vi "Build Variability Plot from Reference.vi"(4 "Group Cols":i32[](array[numeric])=[2], 6 "Y-axis Col":i32=20, 8 "Size of Legend (%)":dbl=0.2, 9 "Column Header Strings":string[](array[string])=["Unique_ID", "Wafer_Name", "Split", "Cell", "Sample_Type", "Experiment", "Active_Area_(cm2)", "Num_of_cell_tests", "Date-Time", "User_Name", "Irradiance_(W/cm2)", "Temperature(C)", "Sweep_Type", "Bulb_Power", "Bulb_Flux(uA)", "Last_Calibrated_Date-Time", "Last_Bulb_Replacement_Date-Time", "Comments", "Unique_ID", "Eff", "Voc_(V)", "Jsc_(A/cm2)", "Fill_Factor", "Roc_(ohm*cm2)", "Rsc_(ohm*cm2)", "Pmax_(W/cm2)", "Vmp_(V)", "Jmp_(A/cm2)", "Model R2", "Dark_Turn-on_V", "Ideality_Factor", "J0_(A/cm2)", "J0_Diffusion_(A/cm2)", "J0_GR_(A/cm2)", "Rsh_(Ohm*cm2)", "Rs_(Ohm*cm2)", "CE_(%)"], 10 "Input Table":string[][](array[string])=[["ID03172011132910", "D11014", "B5", "1", "Crystal CdTe", "CZT EXP009", "0.0143", "2", "3/17/2011 1:29:10 PM", "dtester", "0.1", "25", "Custom - Uses option tab setting", "1155", "161.6", "3/17/2011 1:24:56 PM", "5/25/2010 1:00:00 PM", "", "ID03172011132910", "0.000018331135", "0.329199646", "-0.000019162902", "0.290582012", "12248.694", "23122.247", "0.000001833114", "0.179016841", "0.000010239894", "0", "0.992889686", "8.68126209E-46", "4.422637E-12", "4451299", "-131.960127", "61928.868", "", "", "", "", ""], ["ID03172011133056", "D11014", "B5", "2", "Crystal CdTe", "CZT EXP009", "0.0143", "1", "3/17/2011 1:30:56 PM", "dtester", "0.1", "25", "Custom - Uses option tab setting", "1155", "161.6", "3/17/2011 1:24:56 PM", "5/25/2010 1:00:00 PM", "", "ID03172011133056", "0.000019774033", "0.343694416", "-0.000019403825", "0.29650732", "11605.468", "24816.221", "0.000001977403", "0.188833978", "0.00001047165", "3222.311", "0.992305147", "4.10762544E-46", "4.64417E-12", "5095988", "-116.319344", "80376.492", "", "", "", "", ""], ["ID03172011134450", "D11016", "E4", "1", "Crystal CdTe", "CZT EXP009", "0.0143", "2", "3/17/2011 1:44:50 PM", "dtester", "0.1", "25", "Custom - Uses option tab setting", "0", "161.6", "3/17/2011 1:24:56 PM", "5/25/2010 1:00:00 PM", "", "ID03172011134450", "0", "0.066337846", "-0.000001549743", "0", "24000.955", "355279.503", "0", "0", "0", "0", "0.932694566", "4.712838E-48", "1.521848E-12", "100000000000000", "-1301.062", "361382.131", "", "", "", "", ""], ["ID03172011134552", "D11016", "E4", "2", "Crystal CdTe", "CZT EXP009", "0.0143", "1", "3/17/2011 1:45:52 PM", "dtester", "0.1", "25", "Custom - Uses option tab setting", "0", "161.6", "3/17/2011 1:24:56 PM", "5/25/2010 1:00:00 PM", "", "ID03172011134552", "0.000001609791", "0.18902661", "-0.000004209879", "0.202291173", "55653.293", "29563.168", "0.0000001609791", "0.093729707", "0.000001717482", "0", "0.836775618", "3.606545E-48", "0.000000003769194", "100000000000000", "-504.246188", "546040.796", "", "", "", "", ""], ["ID03172011134725", "D11017", "A3", "1", "Crystal CdTe", "CZT EXP009", "0.0143", "1", "3/17/2011 1:47:25 PM", "dtester", "0.1", "25", "Custom - Uses option tab setting", "0", "161.6", "3/17/2011 1:24:56 PM", "5/25/2010 1:00:00 PM", "", "ID03172011134725", "0.000007862703", "0.300634425", "-0.000009351238", "0.279681693", "25122.784", "37448.672", "0.00000078627026", "0.161786792", "0.000004859916", "0", "0.998501747", "1.881718E-48", "3.03841765E-10", "7111744", "-173.547592", "554111.9", "", "", "", "", ""], ["ID03172011134847", "D11017", "A3", "3", "Crystal CdTe", "CZT EXP009", "0.0143", "1", "3/17/2011 1:48:47 PM", "dtester", "0.1", "25", "Custom - Uses option tab setting", "0", "161.6", "3/17/2011 1:24:56 PM", "5/25/2010 1:00:00 PM", "", "ID03172011134847", "0.000007726846", "0.299639907", "-0.000009106517", "0.283171979", "25227.847", "39025.402", "0.000000772684597", "0.161170617", "0.000004794203", "29301660", "0.996689983", "9.30590943E-49", "8.7875222E-11", "7981629", "-169.139745", "676093.501", "", "", "", "", ""], ["ID03172011135004", "D11016", "E2", "1", "Crystal CdTe", "CZT EXP009", "0.0143", "1", "3/17/2011 1:50:04 PM", "dtester", "0.1", "25", "Custom - Uses option tab setting", "0", "161.6", "3/17/2011 1:24:56 PM", "5/25/2010 1:00:00 PM", "", "ID03172011135004", "0.000008887575", "0.314422094", "-0.000011008741", "0.256763078", "24162.056", "38566.512", "0.000000888757533", "0.135568669", "0.000006555774", "372634.151", "0.99877204", "2.5938593E-47", "1.00830354E-10", "6315776", "-188.727106", "224030.183", "", "", "", "", ""], ["ID03172011135102", "D11016", "E2", "2", "Crystal CdTe", "CZT EXP009", "0.0143", "1", "3/17/2011 1:51:02 PM", "dtester", "0.1", "25", "Custom - Uses option tab setting", "0", "161.6", "3/17/2011 1:24:56 PM", "5/25/2010 1:00:00 PM", "", "ID03172011135102", "0.000008220737", "0.299774635", "-0.000008826217", "0.310700021", "23973.842", "26397.011", "0.000000822073702", "0.180441307", "0.000004555906", "0", "0.998383932", "2.0025352E-47", "1.04854738E-10", "6274781", "-214.846448", "244423.023", "", "", "", "", ""], ["ID03172011135230", "D11017", "C1", "1", "Crystal CdTe", "CZT EXP009", "0.0143", "1", "3/17/2011 1:52:30 PM", "dtester", "0.1", "25", "Custom - Uses option tab setting", "0", "161.6", "3/17/2011 1:24:56 PM", "5/25/2010 1:00:00 PM", "", "ID03172011135230", "0.000009002015", "0.322095736", "-0.000010017559", "0.278992685", "25552.404", "38853.628", "0.000000900201474", "0.172166433", "0.00000522867", "16809035", "0.998577656", "5.83859492E-49", "3.0578151E-10", "7303523", "-156.257879", "798891.399", "", "", "", "", ""], ["ID03172011135446", "D11014", "A2", "1", "Crystal CdTe", "CZT EXP009", "0.0143", "1", "3/17/2011 1:54:46 PM", "dtester", "0.1", "25", "Custom - Uses option tab setting", "0", "161.6", "3/17/2011 1:24:56 PM", "5/25/2010 1:00:00 PM", "retry", "ID03172011135446", "0.000008121558", "0.318938896", "-0.000008607329", "0.295844468", "25228.235", "29753.235", "0.000000812155756", "0.158334247", "0.000005129375", "0", "0.996400609", "2.016331E-48", "3.99575382E-10", "9290112", "-74.919625", "546763.331", "", "", "", "", ""], ["ID03172011135542", "D11014", "A2", "2", "Crystal CdTe", "CZT EXP009", "0.0143", "1", "3/17/2011 1:55:42 PM", "dtester", "0.1", "25", "Custom - Uses option tab setting", "0", "162", "3/17/2011 1:24:56 PM", "5/25/2010 1:00:00 PM", "retry", "ID03172011135542", "0.000010769773", "0.316532242", "-0.000010678727", "0.31861711", "18332.836", "32777.717", "0.000001076977", "0.185023821", "0.000005820749", "0", "0.994541054", "3.879299E-48", "9.0565763E-11", "8933675", "-113.837654", "437235.26", "", "", "", "", ""], ["ID03172011135702", "D11016", "C3", "1", "Crystal CdTe", "CZT EXP009", "0.0143", "1", "3/17/2011 1:57:02 PM", "dtester", "0.1", "25", "Custom - Uses option tab setting", "0", "161.6", "3/17/2011 1:24:56 PM", "5/25/2010 1:00:00 PM", "retry", "ID03172011135702", "0.000005099675", "0.235096132", "-0.000007926189", "0.27367339", "25734.358", "34044.701", "0.000000509967465", "0.123146343", "0.00000414115", "4091317000", "0.989780648", "6.5732986E-50", "0.00000012792339", "6862941", "-258.957329", "1691082", "", "", "", "", ""], ["ID03172011135800", "D11016", "C3", "2", "Crystal CdTe", "CZT EXP009", "0.0143", "1", "3/17/2011 1:58:00 PM", "dtester", "0.1", "25", "Custom - Uses option tab setting", "0", "161.6", "3/17/2011 1:24:56 PM", "5/25/2010 1:00:00 PM", "retry", "ID03172011135800", "0.000006572242", "0.277556032", "-0.00000897193", "0.263922873", "36049.094", "36545.224", "0.000000657224249", "0.14400509", "0.000004563896", "4327975000000", "0.969663856", "1.11030837E-52", "3.012567E-14", "205688100", "-168.692902", "9146911", "", "", "", "", ""]], 11 "Variability Plot Reference":refnum<vi>) -> ()   [LabVIEW 2010]
uses:
  <vilib>/Analysis/NI_AALBase.lvlib
panel:
  out "appended array":cluster{dbl[], dbl[]}[](array[cluster])
  out "subarray":dbl[](array[numeric])
  out "Bottom":dbl=0.010866531999999998
  out "Array":cluster{"String":string, dbl, dbl}[](array[cluster])=[{"String"="A2", 1.0, 0.038602189}, {"String"="A3", 2.0, 0.038602189}, {"String"="B5", 3.0, 0.038602189}, {"String"="C1", 4.0, 0.038602189}, {"String"="C3", 5.0, 0.038602189}, {"String"="E2", 6.0, 0.038602189}, {"String"="E4", 7.0, 0.038602189}]
  out "List of Categories":string[][](array[string])=[["A2"], ["A3"], ["B5"], ["C1"], ["C3"], ["E2"], ["E4"]]
  out "Parameter Analysis Graph":cluster{"Voltage":dbl[], dbl[]}[](graph)=[{"Voltage"=[3.0, 3.0, 7.0, 7.0, 2.0, 2.0, 6.0, 6.0, 4.0, 1.0, 1.0, 5.0, 5.0], [0.329199646, 0.343694416, 0.066337846, 0.18902661, 0.300634425, 0.299639907, 0.314422094, 0.299774635, 0.322095736, 0.318938896, 0.316532242, 0.235096132, 0.277556032]}, {"Voltage"=[1.0, 2.0, 3.0, 4.0, 5.0, 6.0, 7.0], [0.317735569, 0.30013716599999996, 0.336447031, 0.322095736, 0.256326082, 0.3070983645, 0.127682228]}, {"Voltage"=[0.0, 8.0, 8.0, 0.0], [0.010866531999999998, 0.010866531999999998, 0.066337846, 0.066337846]}, {"Voltage"=[0.5, 0.5], [0.066337846, inf]}]
  # "Most General"
  # "Most Specific"
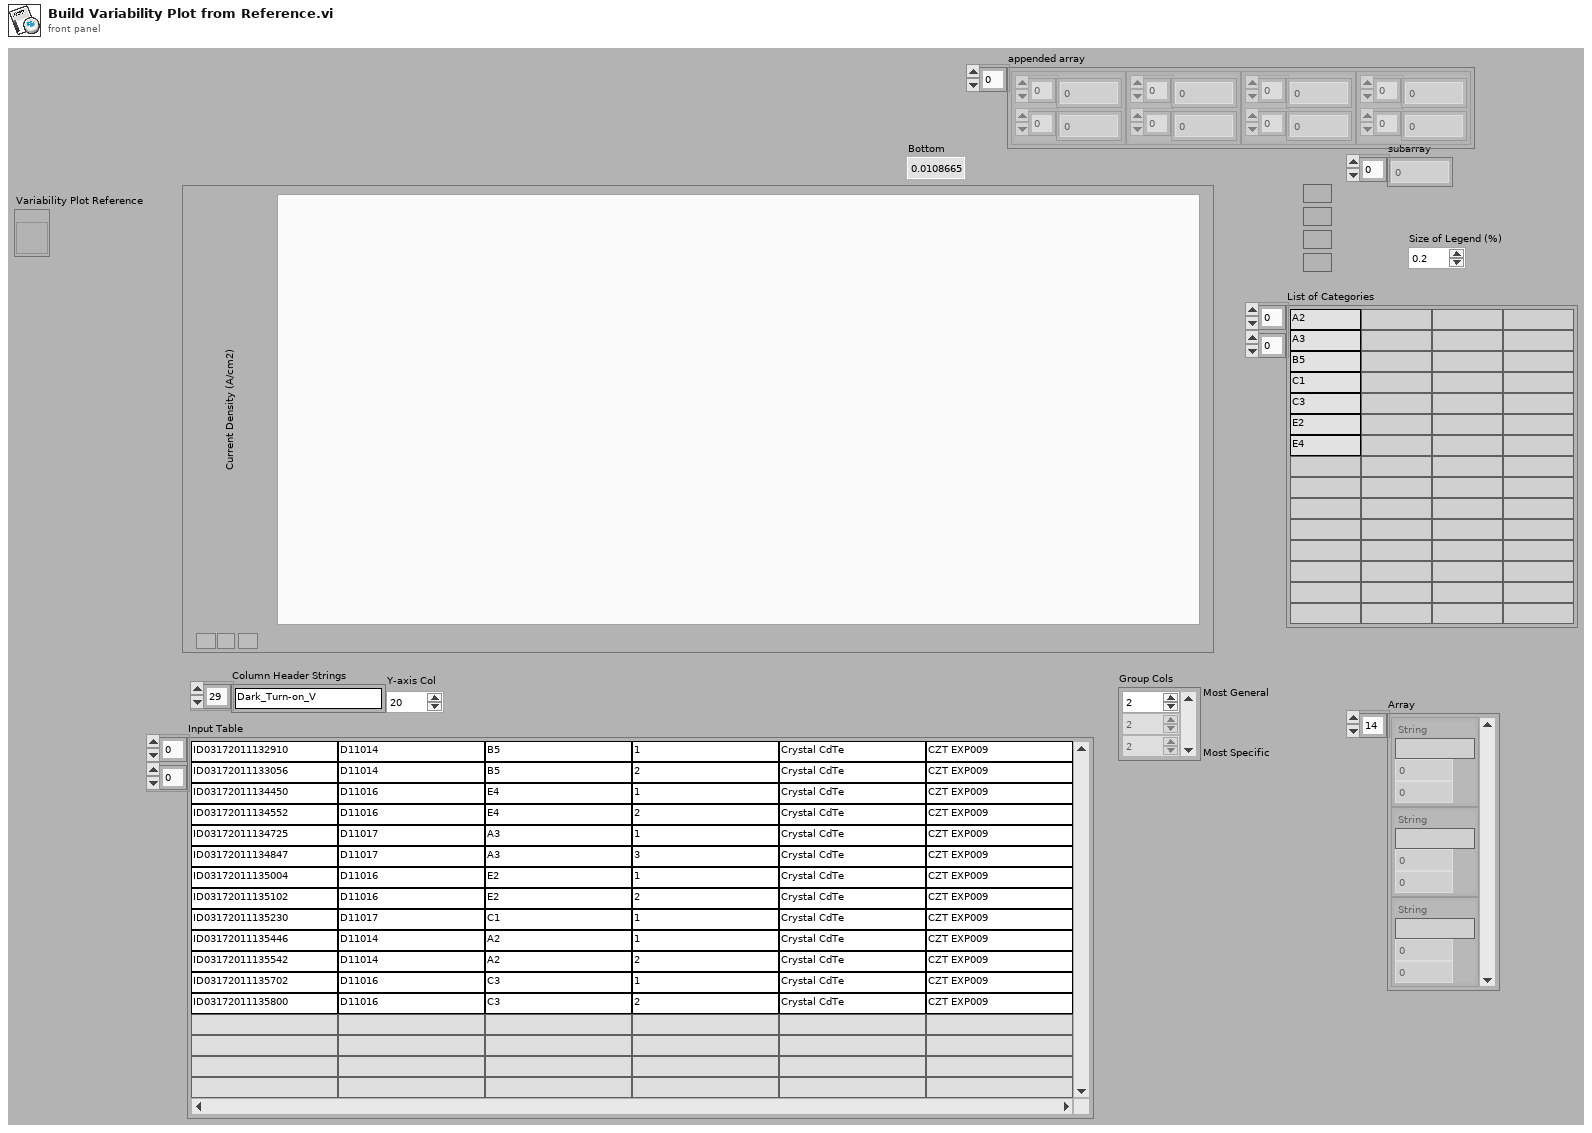
[diagram p1: front panel]
types:
  T1 = cluster{"Name":string, "Color":u32, "Style":u8, "Point Style":u8, "Name Visible":bool, "Allow Drag":bool, "Annotation Mode":u32, "Plot":i32, "Index":i32, "Position":cluster{"X":dbl, "Y":dbl}, "X Scale":u32, "Y Scale":u32, "Show Arrow":bool, "Lock Name":bool, "Plot Area":i32, "Label Offset":cluster{"X":dbl, "Y":dbl}}
  T2 = cluster{"Name":string, "Color":u32, "Style":u8, "Point Style":u8, "Name Visible":bool, "Allow Drag":bool, "Annotation Mode":u32, "Plot":i32, "Index":i32, "Position":cluster{"X":dbl, "Y":dbl}, "X Scale":u32, "Y Scale":u32, "Show Arrow":bool, "Lock Name":bool, "Plot Area":i32, "Label Offset":cluster{"X":dbl, "Y":dbl}}[]
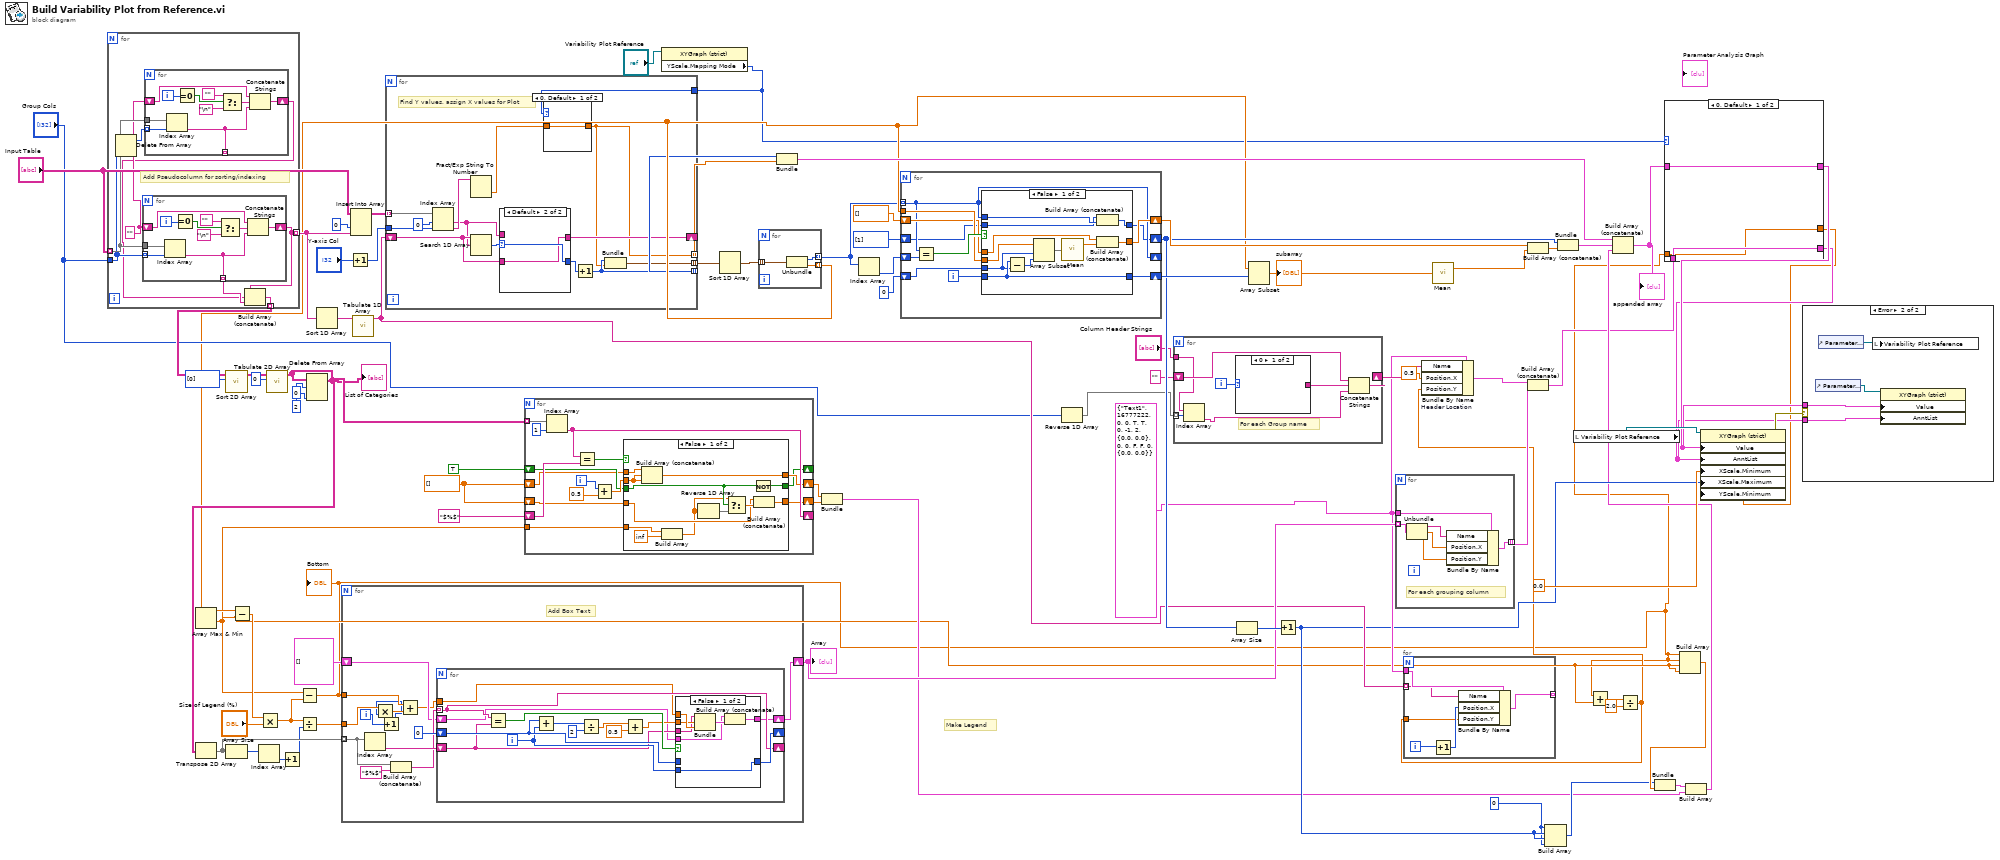
[diagram p0: block diagram]
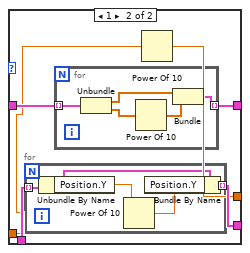
[diagram p2: hidden frame]
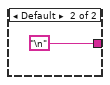
[diagram p6: hidden frame]
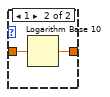
[diagram p8: hidden frame]
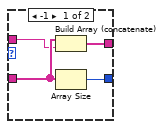
[diagram p9: hidden frame]
diagram:
  w27 = 0
  w46 = dbl[] []
  w29 = T1 {"Name"="Text1", "Color"=16777222, "Style"=0, "Point Style"=0, "Name Visible"=TRUE, "Allow Drag"=TRUE, "Annotation Mode"=0, "Plot"=-1, "Index"=2, "Position"={"X"=0.0, "Y"=0.0}, "X Scale"=0, "Y Scale"=0, "Show Arrow"=FALSE, "Lock Name"=FALSE, "Plot Area"=0, "Label Offset"={"X"=0.0, "Y"=0.0}} ("element")
  # "Make Legend"
  n1 = for {
    tunnel: "Input Table" -> [w87] mode=indexing
    tunnel: "Group Cols" -> [w85]
    tunnel: [w90] -> w64 mode=indexing
    tunnel: [w88] -> w52 mode=indexing
    w86 = ""
    # "Add Pseudocolumn for sorting/indexing"
    n2 = Delete From Array(array=w85) -> (array with subset deleted=w84:i32[])  [unwired: 2 in, 1 out]
    n3 = for {
      tunnel: w85 -> [w109] mode=indexing
      tunnel: w87 -> [w110]
      shift-right: [w108] -> w90
      shift-left: w86 -> [w107]
      tunnel: [w101] -> w89 mode=indexing
      i -> [w105]
      n4 = Index Array(array=w110, index=w109) -> (element=w101:string)
      n5 = Equal To 0?(x=w105) -> (x = 0?=w106:bool)
      n6 = Select(t="", s=w106, f="\n") -> (s? t:f=w102:string)
      n7 = Concatenate Strings(w107, w102, w101) -> (w108:string)
    }
    n8 = for {
      tunnel: w84 -> [w99] mode=indexing
      tunnel: w87 -> [w100]
      shift-right: [w98] -> w83
      shift-left: w86 -> [w97]
      tunnel: [w91] -> _ mode=indexing
      i -> [w95]
      n9 = Index Array(array=w100, index=w99) -> (element=w91:string)
      n10 = Equal To 0?(x=w95) -> (x = 0?=w96:bool)
      n11 = Select(t="", s=w96, f="\n") -> (s? t:f=w92:string)
      n12 = Concatenate Strings(w97, w92, w91) -> (w98:string)
    }
    n13 = Build Array (concatenate)(w90, w83, w89) -> (w88:string[])
  }
  n14 = call "Sort 2D Array.vi"("Sort by Cols"=i32[] [0], "Input Array"=w52) -> ("Output Array"=w55:string[][])  [unwired: 9 in]
  n15 = call "Tabulate 2D Array.vi"("Tabulation Column"=0, "Input Array"=w55) -> ("Tabulation"=w42:string[][])  [unwired: 9 in]
  n16 = Delete From Array(array=w42, length=2, index (col)=0 ("index (row)")) -> (array with subset deleted=w41:string[][])  [unwired: 1 in, 1 out]
  "List of Categories" <- w41
  n17 = Transpose 2D Array(2D array=w41) -> (transposed array=w34:string[][])
  n18 = Array Size(array=w34) -> (size(s)=w33:i32[])
  n19 = Index Array(array=w33) -> (element=w20:i32)  [unwired: 1 in]
  n20 = Increment(x=w20) -> (x+1=w19:i32)
  n21 = Sort 1D Array(array=w64) -> (sorted array=w67:string[])
  n22 = Increment(x="Y-axis Col") -> (x+1=w63:i32)
  n23 = Insert Into Array(array="Input Table", index (col)=0 ("disabled index (col)"), new element=w64) -> (w57:string[][])  [unwired: 1 in]
  n24 = call "Tabulate 1D Array.vi"("1D Array"=w67) -> ("Tabulated Array"=w39:string[])  [unwired: 10 in]
  n25 = property class="XYGraph (strict)"(reference="Variability Plot Reference") -> ("YScale.Mapping Mode"=w1:u8)  [unwired: 1 in, 2 out]
  n26 = for {
    tunnel: w57 -> [w119] mode=indexing
    shift-right: [w123] -> _
    shift-left: w39 -> [w122]
    tunnel: [w111] -> w2 mode=indexing
    tunnel: [w120] -> w66 mode=indexing
    tunnel: w63 -> [w118]
    tunnel: [w116] -> w3 mode=indexing
    tunnel: w1 -> [w113]
    # "Find Y values, assign X values for Plot"
    n27 = Index Array(array=w119, index #1=0 ("index"), index #2=w118) -> (element #1=w115:string, element #2=w117:string)
    n28 = Fract/Exp String To Number(string=w117) -> (number=w112:dbl)  [unwired: 3 in, 1 out]
    n29 = Search 1D Array(1D array=w122, element=w115) -> (index of element=w124:i32)  [unwired: 1 in]
    n30 = case shown="Default" w124 {
      selector: w124 -> [_ w133]
      tunnel: w115 -> [w128 _]
      tunnel: [w131 w132] -> w123
      tunnel: w122 -> [w129 w132]
      tunnel: [w130 w133] -> w121
      frame -1 {
        n31 = Build Array (concatenate)(w129, w128) -> (w131:string[])
        n32 = Array Size(array=w129) -> (size(s)=w130:i32)
      }
      frame Default {
      }
    }
    n33 = case shown="0, Default" w113 {
      tunnel: w112 -> [w125 w127]
      tunnel: [w125 w126] -> w111
      frame 0, Default {
      }
      frame 1 {
        n34 = Logarithm Base 10(1:w127) -> (0:w126:dbl)
      }
    }
    n35 = Increment(x=w121) -> (x+1=w116:i32)
    n36 = Bundle(w116, w111) -> (w120:cluster{i32, dbl})  [unwired: 1 in]
  }
  n37 = Sort 1D Array(array=w66) -> (sorted array=w59:cluster{i32, dbl}[])
  n38 = for {
    tunnel: w59 -> [w136] mode=indexing
    tunnel: [w135] -> w4 mode=indexing
    tunnel: [w134] -> w10 mode=indexing
    n39 = Unbundle(w136) -> (w135:i32, w134:dbl)
  }
  n40 = Array Max & Min(array=w10) -> (max value=w30:dbl, min value=w16:dbl)  [unwired: 2 out]
  n41 = Subtract(x=w30, y=w16) -> (x-y=w26:dbl)
  n42 = Multiply(x=w26, y="Size of Legend (%)") -> (x*y=w35:dbl)
  n43 = Subtract(x=w16, y=w35) -> (x-y=w7:dbl)
  "Bottom" <- w7
  n44 = Divide(x=w35, y=w19) -> (x/y=w32:dbl)
  n45 = for {
    tunnel: w34 -> [w147] mode=indexing
    shift-right: [w144] -> w40
    shift-left: cluster{"String":string, dbl, dbl}[] [] -> [w143]
    tunnel: w7 -> [w140]
    tunnel: w32 -> [w139]
    i -> [w138]
    # "Add Box Text"
    n46 = Index Array(array=w147) -> (element=w149:string)  [unwired: 1 in]
    n47 = Increment(x=w138) -> (x+1=w137:i32)
    n48 = Multiply(x=w139, y=w137) -> (x*y=w142:dbl)
    n49 = Build Array (concatenate)(w147, "$%$" ("String")) -> (w145:string[])
    n50 = Add(x=w140, y=w142) -> (x+y=w141:dbl)
    n51 = for {
      tunnel: w145 -> [w155] mode=indexing
      shift-right: [w155] -> _
      shift-left: w149 -> [w153]
      shift-right: [w162] -> _
      shift-left: 0 -> [w158]
      shift-right: [w151] -> w144
      shift-left: w143 -> [w150]
      tunnel: w141 -> [w152]
      i -> [w157]
      n52 = Equal?(x=w155, y=w153) -> (x = y?=w163:bool)
      n53 = Add(x=w158, y=w157) -> (x+y=w156:i32)
      n54 = Divide(x=w156, y=2) -> (x/y=w160:dbl)
      n55 = Add(x=w160, y=0.5) -> (x+y=w154:dbl)
      n56 = case shown="False" w163 {
        tunnel: w157 -> [w170 _]
        tunnel: [w170 w172] -> w162
        tunnel: w158 -> [_ w172]
        tunnel: w154 -> [w168 _]
        tunnel: w152 -> [w169 _]
        tunnel: w153 -> [w167 _]
        tunnel: [w165 w171] -> w151
        tunnel: w150 -> [w164 w171]
        frame False {
          n57 = Bundle("String"=w167, w168, w169) -> (w166:cluster{"String":string, dbl, dbl})  [unwired: 1 in]
          n58 = Build Array (concatenate)(w164, w166) -> (w165:cluster{"String":string, dbl, dbl}[])
        }
        frame True {
        }
      }
    }
  }
  "Array" <- w40
  n59 = for {
    tunnel: w42 -> [w187] mode=indexing
    shift-right: [w186] -> _
    shift-left: "$%$" ("String") -> [w185]
    shift-right: [w179] -> w45
    shift-left: w46 -> [w178]
    shift-right: [w177] -> _
    shift-left: TRUE -> [w180]
    shift-right: [w176] -> w44
    shift-left: w46 -> [w175]
    tunnel: w16 -> [w173]
    i -> [w183]
    n60 = Index Array(array=w187, index=1) -> (element=w186:string)
    n61 = Equal?(x=w186, y=w185) -> (x = y?=w184:bool)
    n62 = Add(x=w183, y=0.5) -> (x+y=w181:dbl)
    n63 = case shown="False" w184 {
      tunnel: w181 -> [w199 _]
      tunnel: w180 -> [w195 w202]
      tunnel: [w197 w200] -> w179
      tunnel: w178 -> [w196 w200]
      tunnel: [w194 w202] -> w177
      tunnel: [w192 w201] -> w176
      tunnel: w175 -> [w191 w201]
      tunnel: w173 -> [w189 _]
      frame False {
        n64 = Build Array (concatenate)(w196, w199, w199) -> (w197:dbl[])
        n65 = Build Array(w189, inf) -> (w188:dbl[])
        n66 = Reverse 1D Array(array=w188) -> (reversed array=w198:dbl[])
        n67 = Select(t=w188, s=w195, f=w198) -> (s? t:f=w193:dbl[])
        n68 = Not(x=w195) -> (.not. x?=w194:bool)
        n69 = Build Array (concatenate)(w191, w193) -> (w192:dbl[])
      }
      frame True {
      }
    }
  }
  n70 = Bundle(w3, w2) -> (w78:cluster{i32[], dbl[]})  [unwired: 1 in]
  n71 = Bundle(w45, w44) -> (w22:cluster{dbl[], dbl[]})  [unwired: 1 in]
  n72 = Index Array(array=w4) -> (element=w82:i32)  [unwired: 1 in]
  n73 = for {
    tunnel: w4 -> [w205] mode=indexing
    tunnel: w10 -> [w208]
    shift-right: [w205] -> _
    shift-left: w82 -> [w213]
    shift-right: [w210] -> w76
    shift-left: 0 -> [w209]
    shift-right: [w207] -> w74
    shift-left: dbl[] [] -> [w206]
    shift-right: [w204] -> w62
    shift-left: i32[] [1] -> [w203]
    i -> [w211]
    n74 = Equal?(x=w205, y=w213) -> (x = y?=w212:bool)
    n75 = case shown="False" w212 {
      tunnel: w211 -> [w223 _]
      tunnel: [w223 w227] -> w210
      tunnel: w209 -> [w222 w227]
      tunnel: w208 -> [w224 _]
      tunnel: [w220 w226] -> w207
      tunnel: w206 -> [w219 w226]
      tunnel: w205 -> [w218 _]
      tunnel: [w217 w225] -> w204
      tunnel: w203 -> [w216 w225]
      frame False {
        n76 = Subtract(x=w223, y=w222) -> (x-y=w221:i32)
        n77 = Array Subset(array=w224, index=w222, length=w221) -> (w215:dbl[])
        n78 = call <vilib>:"Mean.vi"("X"=w215) -> ("mean"=w214:dbl)  [unwired: 1 out]
        n79 = Build Array (concatenate)(w216, w218) -> (w217:i32[])
        n80 = Build Array (concatenate)(w219, w214) -> (w220:dbl[])
      }
      frame True {
      }
    }
  }
  n81 = Reverse 1D Array(array="Group Cols") -> (reversed array=w49:i32[])
  n82 = for {
    shift-right: [w233] -> w72
    shift-left: "" -> [w232]
    tunnel: "Column Header Strings" -> [w230]
    tunnel: w49 -> [w229] mode=indexing
    i -> [w231]
    # "For each Group name"
    n83 = Index Array(array=w230, index=w229) -> (element=w228:string)
    n84 = case shown="0" w231 {
      tunnel: [_ "\n"] -> w234
      frame 0 {
      }
      frame Default {
      }
    }
    n85 = Concatenate Strings(w232, w234, w228) -> (w233:string)
  }
  n86 = Array Size(array=w62) -> (size(s)=w68:i32)
  n87 = Array Subset(array=w10, index=w76) -> (w75:dbl[])  [unwired: 1 in]
  "subarray" <- w75
  n88 = Increment(x=w68) -> (x+1=w28:i32)
  n89 = for {
    tunnel: w29 -> [w241]
    tunnel: [w240] -> w69 mode=indexing
    tunnel: w40 -> [w239] mode=indexing
    # "For each grouping column"
    n90 = Unbundle(w239) -> ("String"=w238:string, w237:dbl, w236:dbl)
    n91 = Bundle By Name(cluster=w241, "Name"=w238, "Position.X"=w237, "Position.Y"=w236) -> (w240:T1)
  }
  n92 = call <vilib>:"Mean.vi"("X"=w75) -> ("mean"=w5:dbl)  [unwired: 1 out]
  n93 = Build Array (concatenate)(w74, w5) -> (w73:dbl[])
  n94 = Build Array(w27, w28, w28, w27) -> (w24:i32[])
  n95 = Bundle(w62, w73) -> (w79:cluster{i32[], dbl[]})  [unwired: 1 in]
  n96 = local read "Variability Plot Reference"() -> (w13:refnum<vi>)
  n97 = Add(x=w7, y=w16) -> (x+y=w18:dbl)
  n98 = Divide(x=w18, y=2.0) -> (x/y=w15:dbl)
  n99 = for {
    tunnel: w39 -> [w246] mode=indexing
    tunnel: w29 -> [w247]
    tunnel: [w243] -> _ mode=indexing
    tunnel: w15 -> [w242]
    i -> [w245]
    n100 = Increment(x=w245) -> (x+1=w244:i32)
    n101 = Bundle By Name(cluster=w247, "Name"=w246, "Position.X"=w244, "Position.Y"=w242) -> (w243:T1)
  }
  n102 = Bundle By Name "Header Location"(cluster=w29, "Name"=w72, "Position.X"=0.5, "Position.Y"=w15) -> (w70:T1)
  n103 = Build Array (concatenate)(w70, w69) -> (w9:T2)
  n104 = Build Array(w7, w7, w16, w16) -> (w25:dbl[])
  n105 = Bundle(w24, w25) -> (w23:cluster{i32[], dbl[]})  [unwired: 1 in]
  n106 = Build Array(w23, w22) -> (w21:cluster{dbl[], dbl[]}[])
  n107 = Build Array (concatenate)(w78, w79, w21) -> (w12:cluster{dbl[], dbl[]}[])
  "appended array" <- w12
  n108 = case shown="0, Default" w1 {
    tunnel: w12 -> [w250 w256]
    tunnel: [w250 w255] -> w11
    tunnel: w9 -> [w249 w254]
    tunnel: [w249 w253] -> w8
    tunnel: w7 -> [w248 w252]
    tunnel: [w248 w251] -> w6
    frame 0, Default {
    }
    frame 1 {
      n109 = for {
        tunnel: w254 -> [w260] mode=indexing
        tunnel: [w259] -> w253 mode=indexing
        n110 = Unbundle By Name(w260) -> ("Position.Y"=w258:dbl)
        n111 = Power Of 10(x=w258) -> (10^x=w257:dbl)
        n112 = Bundle By Name(cluster=w260, "Position.Y"=w257) -> (w259:T1)
      }
      n113 = for {
        tunnel: w256 -> [w265] mode=indexing
        tunnel: [w261] -> w255 mode=indexing
        n114 = Unbundle(w265) -> (w263:dbl[], w264:dbl[])
        n115 = Power Of 10(x=w264) -> (10^x=w262:dbl[])
        n116 = Bundle(w263, w262) -> (w261:cluster{dbl[], dbl[]})  [unwired: 1 in]
      }
      n117 = Power Of 10(x=w252) -> (10^x=w251:dbl)
    }
  }
  n118 = property on="Property Node" class="XYGraph (strict)"(reference=w13, "Value"=w11, "AnntList"=w8, "XScale.Minimum"=0.0 ("X Scale.Range:Minimum"), "XScale.Maximum"=w28, "YScale.Minimum"=w6) -> (error out=w58:errorcluster)  [unwired: 1 in, 1 out]
  n119 = case shown="Error" w58 {
    tunnel: w11 -> [_ w268]
    tunnel: w8 -> [_ w267]
    frame No Error {
    }
    frame Error {
      n120 = control-ref of="Parameter Analysis Graph"() -> (w269:refnum<vi>)
      n121 = control-ref of="Parameter Analysis Graph"() -> (w266:refnum<vi>)
      n122 = local write "Variability Plot Reference"(w266) -> ()
      n123 = property on="Property Node" class="XYGraph (strict)"(reference=w269, "Value"=w268, "AnntList"=w267) -> ()  [unwired: 1 in, 2 out]
    }
  }
